vi "get_number_A.vi"(8 "error in (no error)":errorcluster, 11 "A_Actor in":refnum<class "A_Actor.lvclass">) -> (0 "error out":errorcluster, 3 "A_Actor out":refnum<class "A_Actor.lvclass">)   [LabVIEW 2025, in "A_Actor.lvlib" / "A_Actor.lvclass"]
uses:
  A_Actor.lvclass
  A_Actor.lvclass/A_Actor.ctl
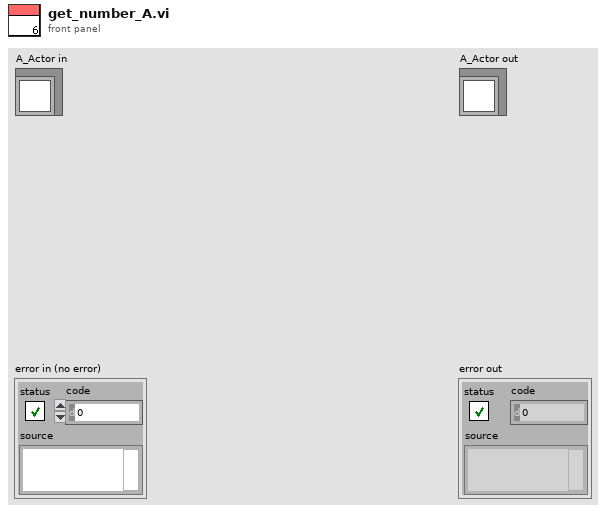
[diagram p1: front panel]
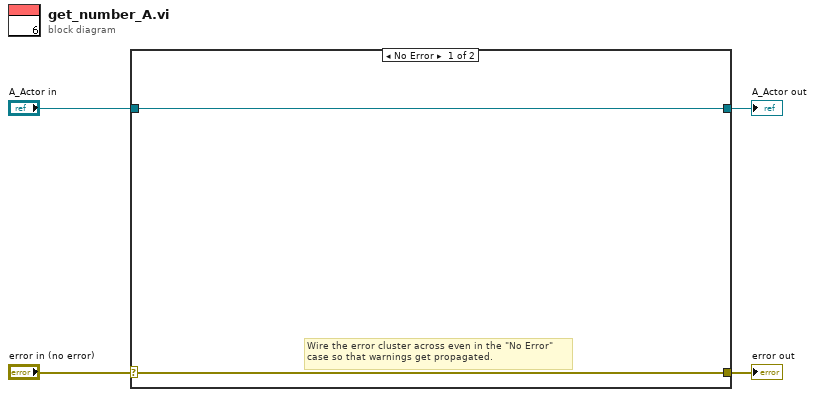
[diagram p0: block diagram]
diagram:
  n1 = case shown="No Error" "error in (no error)" {
    selector: "error in (no error)" -> [w5 w8]
    tunnel: [w5 w8] -> w3
    tunnel: [w6 w7] -> w1
    tunnel: "A_Actor in" -> [w6 w7]
    frame No Error {
      # "Wire the error cluster across even in the \"No Error\"\ncase so that warnings get propagated."
    }
    frame Error {
    }
  }
  "error out" <- w3
  "A_Actor out" <- w1
